vi "JKISM+ TopMain2.vi"() -> ()   [LabVIEW 2014]
uses:
  user.lib/_NEVSTOP/JKI State Machine ++/JKI-State-Machine-Plus.lvlib
panel:
  out "Arguments 3":string
  out "Arguments 2":string
  out "Arguments":string
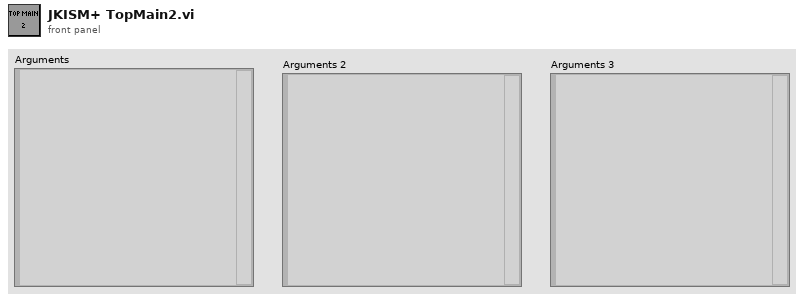
[diagram p1: front panel]
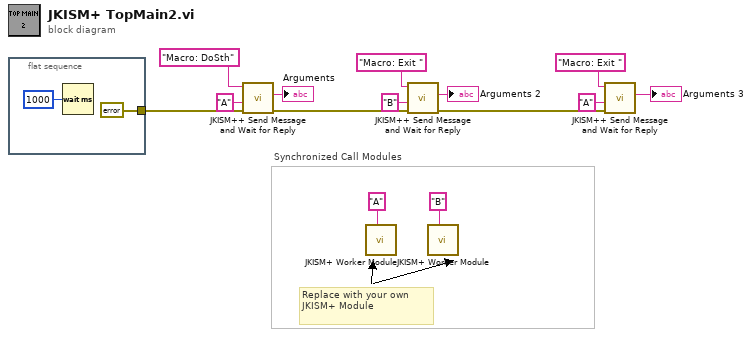
[diagram p0: block diagram]
diagram:
  # "Synchronized Call Modules"
  # "Replace with your own JKISM+ Module"
  n1 = flat-sequence {
    tunnel: [errorcluster {"status"=FALSE, "code"=0, "source"=""} ("Error In (no error)")] -> w4
    frame #0 {
      n2 = Wait (ms)(milliseconds to wait=u32 1000) -> ()  [unwired: 1 out]
    }
  }
  n3 = call "JKISM++ Send Message and Wait for Reply.vi"("Error In (no error)"=w4, "Dest Module"="A", "States"="Macro: DoSth" ("State(s) in Front (\"\")")) -> ("error IO"=w11:errorcluster, "Arguments"=→"Arguments":string)  [unwired: 7 in]
  n4 = call "JKISM+ Worker Module.vi"("Name"="A") -> ()  [unwired: 11 in]
  n5 = call "JKISM++ Send Message and Wait for Reply.vi"("Error In (no error)"=w11, "Dest Module"="B", "States"="Macro: Exit ") -> ("error IO"=w5:errorcluster, "Arguments"=→"Arguments 2":string)  [unwired: 7 in]
  n6 = call "JKISM+ Worker Module.vi"("Name"="B") -> ()  [unwired: 11 in]
  n7 = call "JKISM++ Send Message and Wait for Reply.vi"("Error In (no error)"=w5, "Dest Module"="A", "States"="Macro: Exit ") -> ("Arguments"=→"Arguments 3":string)  [unwired: 7 in, 1 out]
